vi "Inverse Step 3 (SubVI).vi"(0 "Ldist":dbl, 1 "Rdist":dbl, 2 "aLB":dbl, 3 "aRB":dbl, 4 "aLB1":dbl, 5 "aRB1":dbl, 6 "aLB2":dbl, 7 "aRB2":dbl) -> (20 "lcx1":dbl, 21 "lcy1":dbl, 22 "rcx1":dbl, 23 "rcy1":dbl, 24 "aLB1+aLB2":dbl, 25 "aRB1+aRB2":dbl)   [LabVIEW 2015]
uses:
  <vilib>/express/express arith-compare/Formula/XNode/ExpressFormulaBlockNode.xnode
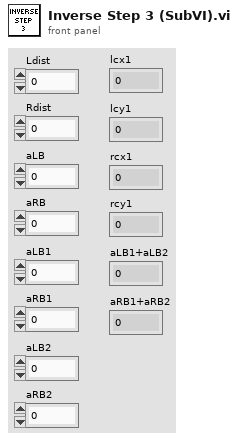
[diagram p1: front panel]
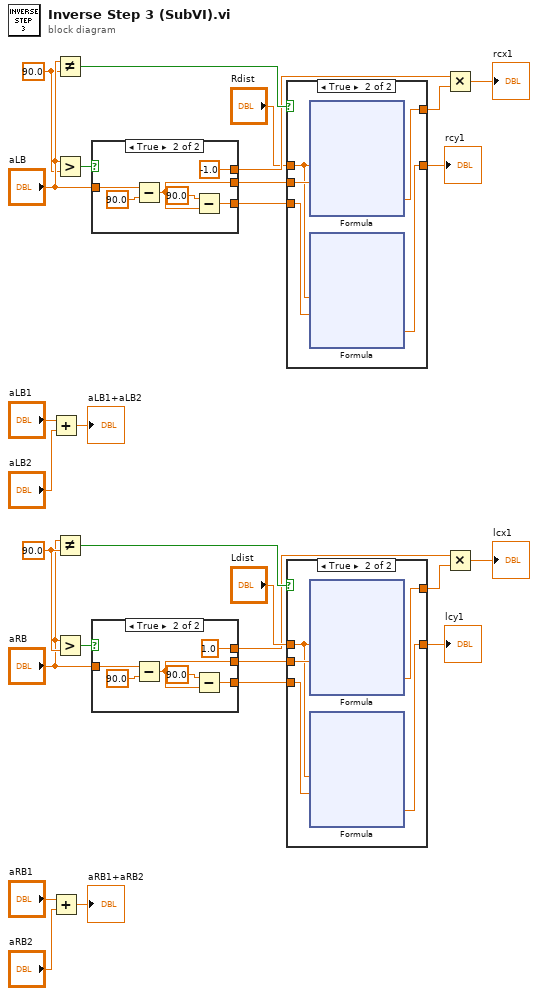
[diagram p0: block diagram]
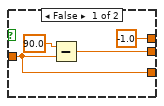
[diagram p2: hidden frame]
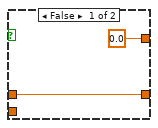
[diagram p3: hidden frame]
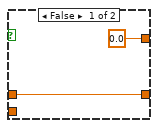
[diagram p4: hidden frame]
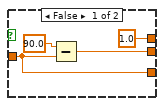
[diagram p5: hidden frame]
diagram:
  w17 = 90.0 ("y")
  w18 = 90.0 ("y")
  n1 = Add(x="aLB1", y="aLB2") -> (x+y=→"aLB1+aLB2":dbl)
  n2 = Add(x="aRB1", y="aRB2") -> (x+y=→"aRB1+aRB2":dbl)
  n3 = Not Equal?(x="aLB", y=w18) -> (x != y?=w21:bool)
  n4 = Greater?(x="aLB", y=w18) -> (0:w22:bool)
  n5 = Not Equal?(x="aRB", y=w17) -> (x != y?=w20:bool)
  n6 = Greater?(x="aRB", y=w17) -> (0:w2:bool)
  n7 = case shown="True" w22 {
    tunnel: "aLB" -> [w30 w38]
    tunnel: [w31 w35] -> w15
    tunnel: [w30 w34] -> w16
    tunnel: [1.0 -1.0] -> w8
    frame False {
      n8 = Subtract(x=90.0, y=w30) -> (x-y=w31:dbl)
    }
    frame True {
      n9 = Subtract(x=w38, y=90.0) -> (x-y=w35:dbl)
      n10 = Subtract(x=90.0, y=w35) -> (x-y=w34:dbl)
    }
  }
  n11 = case shown="True" w2 {
    tunnel: "aRB" -> [w40 w48]
    tunnel: [w41 w45] -> w12
    tunnel: [w40 w44] -> w13
    tunnel: [-1.0 1.0] -> w4
    frame False {
      n12 = Subtract(x=90.0, y=w40) -> (x-y=w41:dbl)
    }
    frame True {
      n13 = Subtract(x=w48, y=90.0) -> (x-y=w45:dbl)
      n14 = Subtract(x=90.0, y=w45) -> (x-y=w44:dbl)
    }
  }
  n15 = case shown="True" w21 {
    tunnel: w16 -> [_ w55]
    tunnel: w15 -> [_ w54]
    tunnel: [0.0 ("Result") w53] -> w9
    tunnel: [w50 w52] -> w7
    tunnel: "Rdist" -> [w50 w51]
    frame False {
    }
    frame True {
      n16 = xnode "Formula"("Ldist"=w51, "aLX"=w54) -> ("Result"=w53:dbl)  [unwired: 1 in, 1 out]
      n17 = xnode "Formula"("Ldist"=w51, "aLY"=w55) -> ("Result"=w52:dbl)  [unwired: 1 in, 1 out]
    }
  }
  "rcy1" <- w7
  n18 = case shown="True" w20 {
    tunnel: w13 -> [_ w82]
    tunnel: w12 -> [_ w81]
    tunnel: [0.0 ("Result") w80] -> w3
    tunnel: [w77 w79] -> w10
    tunnel: "Ldist" -> [w77 w78]
    frame False {
    }
    frame True {
      n19 = xnode "Formula"("Rdist"=w78, "aRX"=w81) -> ("Result"=w80:dbl)  [unwired: 1 in, 1 out]
      n20 = xnode "Formula"("Rdist"=w78, "aRY"=w82) -> ("Result"=w79:dbl)  [unwired: 1 in, 1 out]
    }
  }
  "lcy1" <- w10
  n21 = Multiply(x=w8, y=w9) -> (x*y=→"rcx1":dbl)
  n22 = Multiply(x=w4, y=w3) -> (x*y=→"lcx1":dbl)
